vi "Makerhub Linx Arduino.vi"() -> ()   [LabVIEW 2015]
uses:
  <vilib>/MakerHub/LINX/Public/Peripherals/Digital/Digital Write N Chans.vi
  <vilib>/MakerHub/LINX/Public/Peripherals/Analog/Analog Read N Chans.vi
  <vilib>/MakerHub/LINX/Private/Local IO/LinxDigitalWrite.vi
  <vilib>/MakerHub/LINX/Public/Utilities/Check Channel.vi
  <vilib>/MakerHub/LINX/Private/Local IO/LinxAnalogRead.vi
  <vilib>/MakerHub/LINX/Public/Utilities/Open Serial.vi
  <vilib>/MakerHub/LINX/Private/Utilties/Generate Error.vi
  <vilib>/MakerHub/LINX/LMH-LINX.lvlib
panel:
  out "MQ-5":dbl(slide) scale=0.0..1023.0
  out "LDR":dbl(knob) scale=0.0..1023.0
  out "?":bool
  in  "Values":bool[](array[boolean])
  out "LDR in Voltage":dbl
  out "MQ-5":dbl
  out "LDR":dbl
  out "Voltages":dbl[](array[numeric])
  in  "stop":bool
  out "Device Name":string
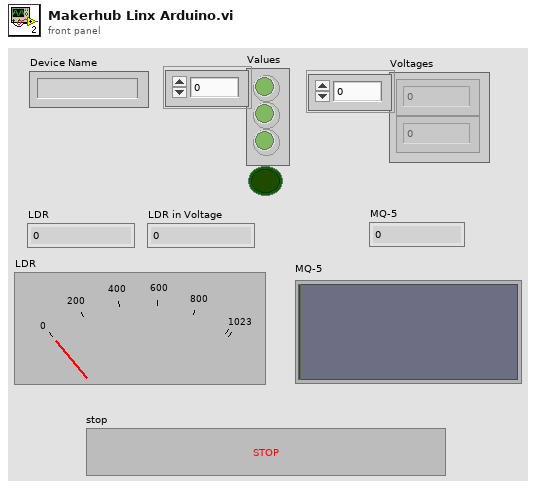
[diagram p1: front panel]
types:
  T1 = typedef "LMH-LINX.lvlib/LINX Ref.ctl" = cluster{"IO":T2, "Interface":T3, "LINX Device Config":T4}
  T2 = typedef "LMH-LINX.lvlib/Platform.ctl" = enum16{"Remote", "Local"}
  T3 = typedef "LMH-LINX.lvlib/Interface.ctl" = enum16{"Serial", "TCP"}
  T4 = typedef "LMH-LINX.lvlib/Device.lvlib/LINX Device Config.ctl" = cluster{"Interface":T3, "COM Port":refnum<visa-resource-name>, "TCP Configuration":T5, "Device Family":u8, "Device ID":u8, "Device Name":string, "TCP Ref":refnum<k5>, "Channels":T6}
  T5 = typedef "LMH-LINX.lvlib/Device.lvlib/TCP Config.ctl" = cluster{"IP Address":string, "Port":u16}
  T6 = typedef "LMH-LINX.lvlib/Channels.ctl" = cluster{"DI":u8[], "DO":u8[], "AI":u8[], "AO":u8[], "PWM":u8[], "QE":u8[], "UART":u8[], "I2C 2":u8[], "SPI":u8[], "CAN":u8[], "Servo":u8[], "AI Ref (V)":dbl, "AI Resolution (Bits)":u8, "AO Ref (V)":dbl, "AO Resolution (Bits)":u8}
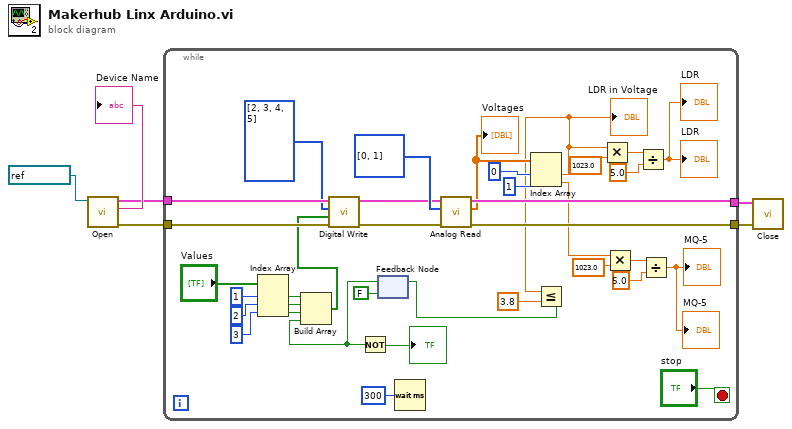
[diagram p0: block diagram]
diagram:
  n1 = call-poly <vilib>:"Open.vi"("Serial Port"=refnum<visa-resource-name> "COM7") -> ("Error Out"=w3:errorcluster, "Device Name"=→"Device Name":string, "LINX Resource"=w5:T1)  [unwired: 8 in]
  n2 = while {
    tunnel: w5 -> [w42]
    tunnel: [w36] -> w4
    tunnel: w3 -> [w41]
    tunnel: [w35] -> w2
    stop <- "stop" stop-if-true
    n3 = Index Array(array="Values", index #1=1 ("index"), index #2=2 ("index"), index #3=3 ("index")) -> (element #1=w14:bool, element #2=w13:bool, element #3=w12:bool)
    n4 = feedback #1(FALSE) -> (w10:bool)
    n5 = Build Array(w14, w13, w12, w10) -> (w11:bool[])
    n6 = call-poly <vilib>:"Digital Write.vi"("Error In"=w41, "Values"=w11, "DO Channels"=i32[] [2, 3, 4, 5], "LINX Resource"=w42) -> ("Error Out"=w38:errorcluster, "LINX Resource"=w37:T1)  [unwired: 6 in]
    n7 = Not(x=w10) -> (.not. x?=→"?":bool)
    n8 = Wait (ms)(milliseconds to wait=u32 300) -> ()  [unwired: 1 out]
    n9 = call-poly <vilib>:"Analog Read.vi"("Error In"=w38, "AI Channel(s)"=u8[] [0, 1] ("Analog Channel"), "LINX Resource"=w37) -> ("Error Out"=w35:errorcluster, "Voltages"=w34:dbl[], "LINX Resource"=w36:T1)  [unwired: 5 in, 1 out]
    "Voltages" <- w34
    n10 = Index Array(array=w34, index #1=0 ("index"), index #2=1 ("index")) -> (element #1=w22:dbl, element #2=w25:dbl)
    "LDR in Voltage" <- w22
    n11 = Less Or Equal?(x=w22, y=3.8) -> (x <= y?=w20:bool)
    n12 = feedback-in #1(w20) -> ()
    n13 = Multiply(x=w22, y=1023.0) -> (x*y=w30:dbl)
    n14 = Multiply(x=w25, y=1023.0) -> (x*y=w27:dbl)
    n15 = Divide(x=w30, y=5.0) -> (x/y=→"LDR" →"LDR":dbl)
    n16 = Divide(x=w27, y=5.0) -> (x/y=→"MQ-5" →"MQ-5":dbl)
  }
  n17 = call <vilib>:"Close.vi"("Error In"=w2, "LINX Resource"=w4) -> ()  [unwired: 9 in, 1 out]
